vi "Get Set Hostname.vi"(8 "Error In":errorcluster, 9 "Set":bool, 10 "Hostname":string, 11 "Install LV Data":T1={"SSH Session"=refnum, "Status Log"="", "Detailed Log"="", "Credentials"={"Hostname or IP"="192.168.7.2", "Username"="root", "Password"=""}, "Target Info"={"OS Version"="", "CPU"="", "Systemd Version"="", "Internet Access"=FALSE, "Device Type"="", "LV Installed Ver"="", "LV Available Ver"="", "LV Upgrade Available"=FALSE, "Hostname"="", "NIC Info"=[]}, "Reboot Required?"=FALSE}) -> (0 "Error Out":errorcluster, 2 "Hostname":string, 3 "Install LV Data":T1={"SSH Session"=refnum, "Status Log"="", "Detailed Log"="", "Credentials"={"Hostname or IP"="192.168.7.2", "Username"="root", "Password"=""}, "Target Info"={"OS Version"="", "CPU"="", "Systemd Version"="", "Internet Access"=FALSE, "Device Type"="", "LV Installed Ver"="", "LV Available Ver"="", "LV Upgrade Available"=FALSE, "Hostname"="", "NIC Info"=[]}, "Reboot Required?"=FALSE})   [LabVIEW 2011, in "LMH-LINX.lvlib"]
uses:
  LMH-LINX.lvlib
  Install LV Data.ctl
  C:/Users/samkristoff/Desktop/Builds/2016_01_27/build/LabVIEW/vi.lib/MakerHub/LINX/Resources/Renci.SshNet.dll
  Resources/Renci.SshNet.dll
  Target Info.ctl
  NIC Info.ctl
  NIC Mode.ctl
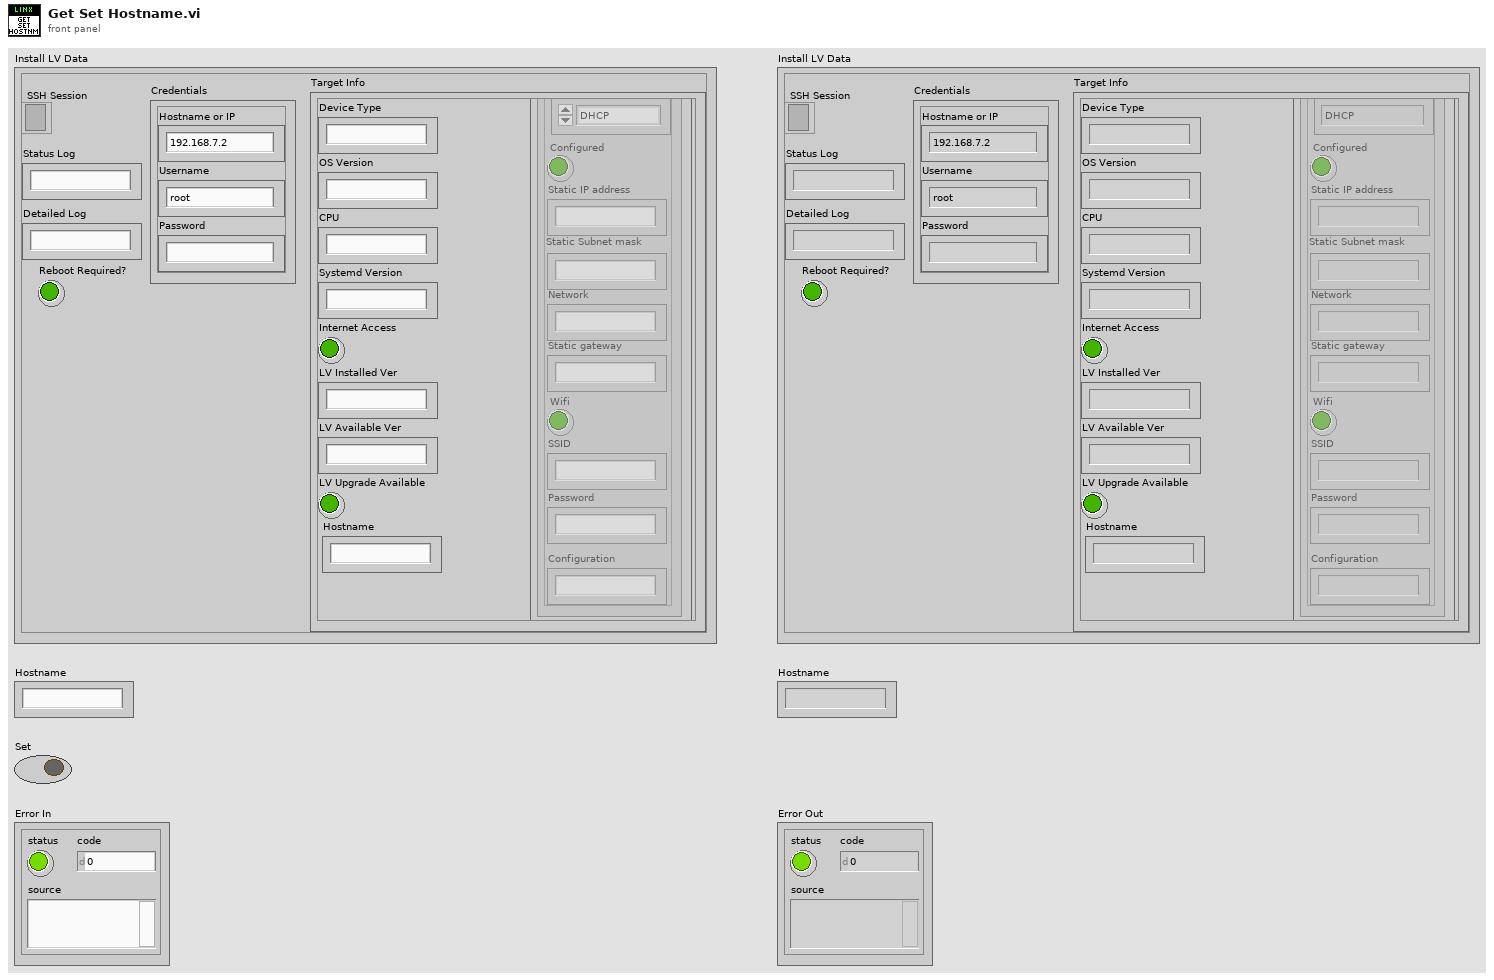
[diagram p1: front panel]
types:
  T1 = typedef "LMH-LINX.lvlib/Install LV Data.ctl" = cluster{"SSH Session":refnum<k24>, "Status Log":string, "Detailed Log":string, "Credentials":cluster{"Hostname or IP":string, "Username":string, "Password":string}, "Target Info":T2, "Reboot Required?":bool}
  T2 = typedef "LMH-LINX.lvlib/Target Info.ctl" = cluster{"OS Version":string, "CPU":string, "Systemd Version":string, "Internet Access":bool, "Device Type":string, "LV Installed Ver":string, "LV Available Ver":string, "LV Upgrade Available":bool, "Hostname":string, "NIC Info":T3[]}
  T3 = typedef "LMH-LINX.lvlib/NIC Info.ctl" = cluster{"Name":string, "NIC Mode":T4, "Configured":bool, "Static IP address":string, "Static Subnet mask":string, "Network":string, "Static gateway":string, "Wifi":bool, "SSID":string, "Password":string, "Configuration":string}
  T4 = typedef "LMH-LINX.lvlib/NIC Mode.ctl" = enum16{"DHCP", "Static", "Loopback"}
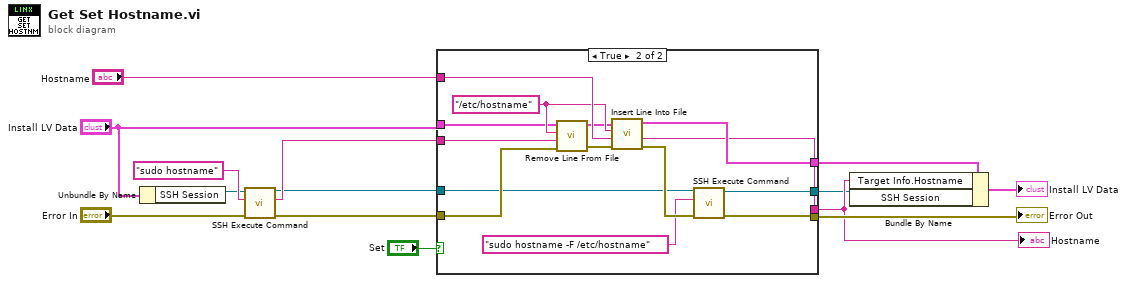
[diagram p0: block diagram]
diagram:
  n1 = Unbundle By Name("Install LV Data") -> ("SSH Session"=w9:refnum<k24>)
  n2 = call "SSH Execute Command.vi"("Error In"="Error In", "Command"="sudo hostname", "SSH Session"=w9) -> ("Error Out"=w12:errorcluster, "Std Out"=w7:string, "SSH Session"=w2:refnum<k24>)  [unwired: 6 in]
  n3 = case shown="True" "Set" {
    tunnel: "Hostname" -> [_ w32]
    tunnel: [w15 w31] -> w6
    tunnel: [w18 w22] -> w13
    tunnel: w7 -> [w17 w27]
    tunnel: w12 -> [w18 w26]
    tunnel: [w17 w25] -> w5
    tunnel: "Install LV Data" -> [w15 w24]
    tunnel: w2 -> [w16 w21]
    tunnel: [w16 w20] -> w1
    frame False {
    }
    frame True {
      w30 = "/etc/hostname" ("File Path")
      n4 = call "Remove Line From File.vi"("Error In"=w26, "Line"=w27, "File Path"=w30, "Install LV Data"=w24) -> ("Error Out"=w29:errorcluster, "Install LV Data"=w28:T1)  [unwired: 4 in, 2 out]
      n5 = call "Insert Line Into File.vi"("Error In"=w29, "Line"=w32, "File Path"=w30, "Install LV Data"=w28) -> ("Error Out"=w23:errorcluster, "Log"=w25:string, "Install LV Data"=w31:T1)  [unwired: 4 in, 1 out]
      n6 = call "SSH Execute Command.vi"("Error In"=w23, "Command"="sudo hostname -F /etc/hostname" ("File Path"), "SSH Session"=w21) -> ("Error Out"=w22:errorcluster, "SSH Session"=w20:refnum<k24>)  [unwired: 6 in, 1 out]
    }
  }
  "Hostname" <- w5
  "Error Out" <- w13
  n7 = Bundle By Name(cluster=w6, "Target Info.Hostname"=w5, "SSH Session"=w1) -> (→"Install LV Data":T1)
